vi "subQuatMultiply.vi"(10 "q2":dbl[](array[numeric]), 11 "q1":dbl[](array[numeric])) -> (3 "qResult":dbl[](array[numeric]))   [LabVIEW 2020]
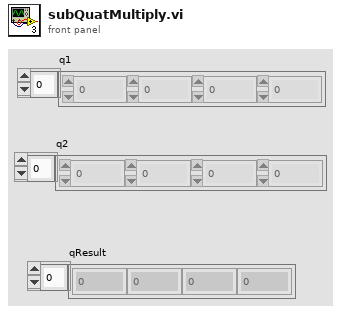
[diagram p1: front panel]
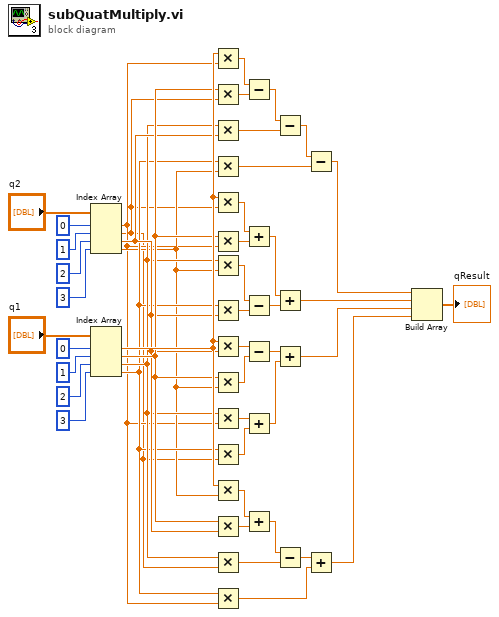
[diagram p0: block diagram]
diagram:
  n1 = Index Array(array="q2", index #1=0, index #2=1, index #3=2, index #4=3) -> (element #1=w2:dbl, element #2=w1:dbl, element #3=w14:dbl, element #4=w3:dbl)
  n2 = Index Array(array="q1", index #1=0, index #2=1, index #3=2, index #4=3) -> (element #1=w16:dbl, element #2=w15:dbl, element #3=w13:dbl, element #4=w12:dbl)
  n3 = Multiply(x=w16, y=w2) -> (x*y=w37:dbl)
  n4 = Multiply(x=w15, y=w1) -> (x*y=w36:dbl)
  n5 = Multiply(x=w13, y=w14) -> (x*y=w34:dbl)
  n6 = Multiply(x=w12, y=w3) -> (x*y=w32:dbl)
  n7 = Multiply(x=w16, y=w1) -> (x*y=w30:dbl)
  n8 = Multiply(x=w15, y=w2) -> (x*y=w29:dbl)
  n9 = Multiply(x=w13, y=w3) -> (x*y=w28:dbl)
  n10 = Multiply(x=w12, y=w14) -> (x*y=w27:dbl)
  n11 = Multiply(x=w16, y=w14) -> (x*y=w23:dbl)
  n12 = Multiply(x=w15, y=w3) -> (x*y=w22:dbl)
  n13 = Multiply(x=w13, y=w2) -> (x*y=w21:dbl)
  n14 = Multiply(x=w12, y=w1) -> (x*y=w20:dbl)
  n15 = Multiply(x=w16, y=w3) -> (x*y=w11:dbl)
  n16 = Multiply(x=w15, y=w14) -> (x*y=w10:dbl)
  n17 = Multiply(x=w13, y=w1) -> (x*y=w8:dbl)
  n18 = Multiply(x=w12, y=w2) -> (x*y=w6:dbl)
  n19 = Subtract(x=w37, y=w36) -> (x-y=w35:dbl)
  n20 = Add(x=w30, y=w29) -> (x+y=w26:dbl)
  n21 = Subtract(x=w28, y=w27) -> (x-y=w25:dbl)
  n22 = Subtract(x=w23, y=w22) -> (x-y=w19:dbl)
  n23 = Add(x=w21, y=w20) -> (x+y=w18:dbl)
  n24 = Add(x=w11, y=w10) -> (x+y=w9:dbl)
  n25 = Subtract(x=w35, y=w34) -> (x-y=w33:dbl)
  n26 = Add(x=w26, y=w25) -> (x+y=w24:dbl)
  n27 = Add(x=w19, y=w18) -> (x+y=w17:dbl)
  n28 = Subtract(x=w9, y=w8) -> (x-y=w7:dbl)
  n29 = Subtract(x=w33, y=w32) -> (x-y=w31:dbl)
  n30 = Add(x=w7, y=w6) -> (x+y=w5:dbl)
  n31 = Build Array(w31, w24, w17, w5) -> (→"qResult":dbl[])
